vi "PZT move.vi"(2 "error in (no error)":errorcluster caption="错误输入（无错误）", 3 "移动步数":i32, 4 "移动方向":u16(ring) items=["正向", "反向"], 5 "VISA resource name":refnum<visa-resource-name> caption="VISA资源名称") -> (0 "错误输出":errorcluster, 1 "VISA资源名称输出":refnum<visa-resource-name>)   [LabVIEW 2019]
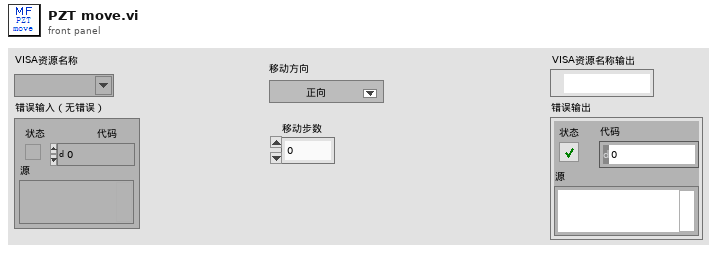
[diagram p1: front panel]
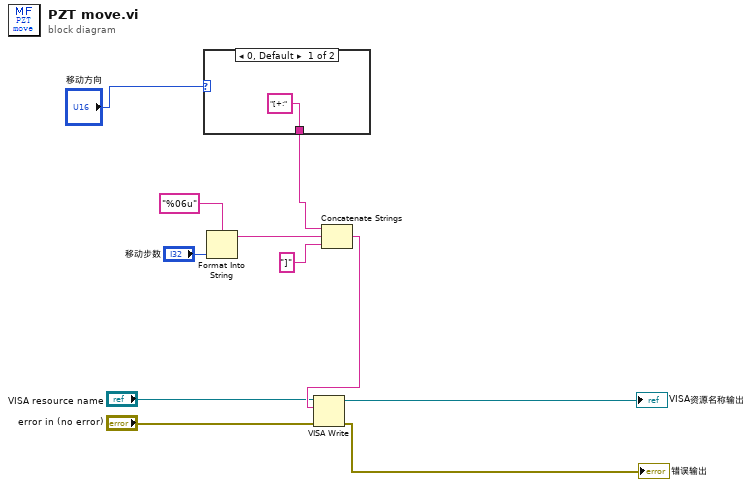
[diagram p0: block diagram]
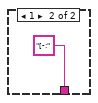
[diagram p2: hidden frame]
diagram:
  n1 = case shown="0, Default" "移动方向" {
    tunnel: ["[+:" ("字符串") "[-:" ("字符串")] -> w4
    frame 0, Default {
    }
    frame 1 {
    }
  }
  n2 = Format Into String(format string="%06u" ("格式字符串"), "移动步数") -> (resulting string=w8:string)  [unwired: 2 in, 1 out]
  n3 = Concatenate Strings(w4, w8, "]" ("字符串")) -> (w6:string)
  n4 = VISA Write(VISA resource name="VISA resource name", write buffer=w6, error in (no error)="error in (no error)") -> (VISA resource name out=→"VISA资源名称输出":refnum<visa-resource-name>, error out=→"错误输出":errorcluster)  [unwired: 1 out]
